vi "MP3 Rename Map.vi"() -> (3 "MP3 Rename Map":map{string, path}(c390))   [LabVIEW 2019, in "Sound.lvlib"]
uses:
  Sound.lvlib
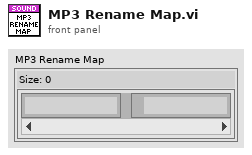
[diagram p1: front panel]
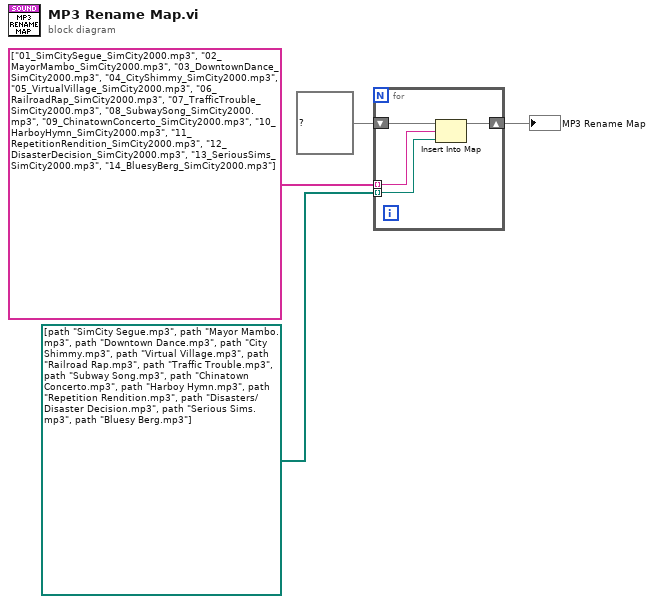
[diagram p0: block diagram]
diagram:
  n1 = for {
    tunnel: string[] ["01_SimCitySegue_SimCity2000.mp3", "02_MayorMambo_SimCity2000.mp3", "03_DowntownDance_SimCity2000.mp3", "04_CityShimmy_SimCity2000.mp3", "05_VirtualVillage_SimCity2000.mp3", "06_RailroadRap_SimCity2000.mp3", "07_TrafficTrouble_SimCity2000.mp3", "08_SubwaySong_SimCity2000.mp3", "09_ChinatownConcerto_SimCity2000.mp3", "10_HarboyHymn_SimCity2000.mp3", "11_RepetitionRendition_SimCity2000.mp3", "12_DisasterDecision_SimCity2000.mp3", "13_SeriousSims_SimCity2000.mp3", "14_BluesyBerg_SimCity2000.mp3"] ("filenames") -> [w8] mode=indexing
    tunnel: path[] [path "SimCity Segue.mp3", path "Mayor Mambo.mp3", path "Downtown Dance.mp3", path "City Shimmy.mp3", path "Virtual Village.mp3", path "Railroad Rap.mp3", path "Traffic Trouble.mp3", path "Subway Song.mp3", path "Chinatown Concerto.mp3", path "Harboy Hymn.mp3", path "Repetition Rendition.mp3", path "Disasters/Disaster Decision.mp3", path "Serious Sims.mp3", path "Bluesy Berg.mp3"] ("path") -> [w7] mode=indexing
    shift-right: [w5] -> w1
    shift-left: map{string, path} {} ("map") -> [w6]
    n2 = Insert Into Map(map in=w6, key=w8, value=w7) -> (map out=w5:map{string, path})  [unwired: 2 out]
  }
  "MP3 Rename Map" <- w1
